vi "Set Property.vi"(8 "error in (no error)":errorcluster, 9 "Value":dbl, 10 "Property":string, 11 "Tone in":refnum<class "Tone.lvclass">) -> (0 "error out":errorcluster, 3 "Tone out":refnum<class "Tone.lvclass">)   [LabVIEW 2020, in "Tone.lvclass"]
uses:
  Tone.lvclass
  Tone.lvclass/Tone.ctl
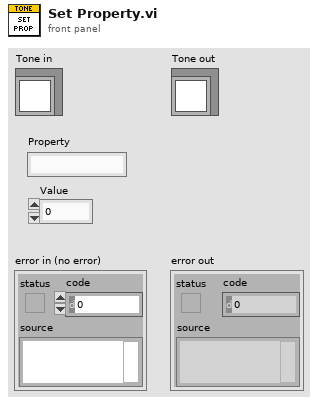
[diagram p1: front panel]
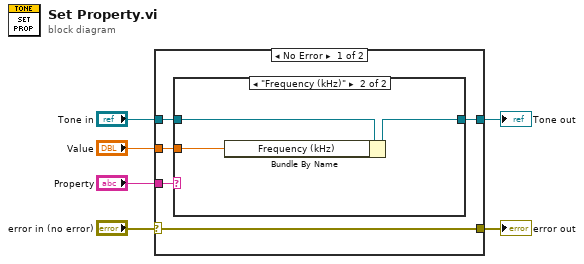
[diagram p0: block diagram]
diagram:
  n1 = case shown="No Error" "error in (no error)" {
    selector: "error in (no error)" -> [w11 w16]
    tunnel: [w11 w16] -> w5
    tunnel: "Property" -> [w10 _]
    tunnel: "Tone in" -> [w9 w17]
    tunnel: "Value" -> [w8 _]
    tunnel: [w7 w17] -> w1
    frame No Error {
      n2 = case shown="\"Frequency (kHz)\"" w10 {
        tunnel: w9 -> [w12 w15]
        tunnel: w8 -> [_ w14]
        tunnel: [w12 w13] -> w7
        frame "", Default {
        }
        frame "Frequency (kHz)" {
          n3 = Bundle By Name(cluster=w15, "Frequency (kHz)"=w14) -> (w13:refnum<class "Tone.lvclass">)
        }
      }
    }
    frame Error {
    }
  }
  "error out" <- w5
  "Tone out" <- w1
